vi "6.2_FileWriter.vi"() -> ()   [LabVIEW 2025]
panel:
  in  "Numeric to Write":dbl
  in  "Unit to Write":string
  in  "String to Write":string
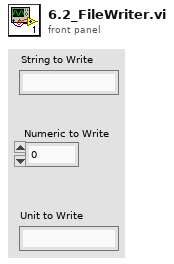
[diagram p1: front panel]
types:
  T1 = enum16{"open", "replace", "create", "open or create", "replace or create", "replace or create with confirmation"}
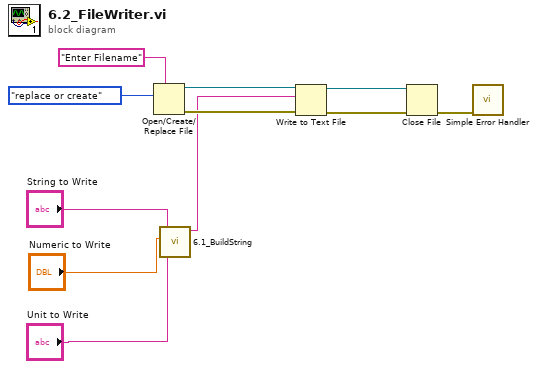
[diagram p0: block diagram]
diagram:
  n1 = Open/Create/Replace File(prompt="Enter Filename", operation (0:open)=T1."replace or create") -> (refnum out=w6:refnum<file>, error out=w4:errorcluster)  [unwired: 4 in, 1 out]
  n2 = call "6.1_BuildString.vi"("Trailer"="Unit to Write", "Numeric"="Numeric to Write", "Header"="String to Write") -> ("Combined String"=w1:string)  [unwired: 1 in, 3 out]
  n3 = Write to Text File(file (use dialog)=w6, text=w1, error in=w4) -> (refnum out=w5:refnum<file>, error out=w3:errorcluster)  [unwired: 1 in, 1 out]
  n4 = Close File(refnum=w5, error in=w3) -> (error out=w2:errorcluster)  [unwired: 1 out]
  n5 = call <vilib>:"Simple Error Handler.vi"("error in (no error)"=w2) -> ()  [unwired: 4 in, 5 out]
